vi "2.1调用.vi"(1 "数值 3":dbl, 2 "数值 2":dbl, 3 "数值":dbl) -> (0 "数值 4":dbl)   [LabVIEW 2017]
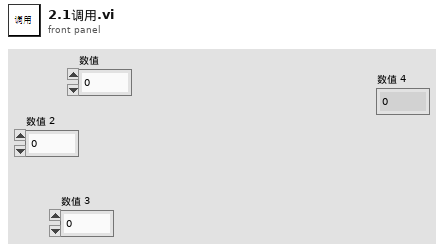
[diagram p1: front panel]
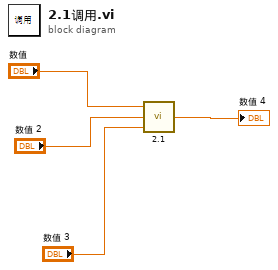
[diagram p0: block diagram]
diagram:
  n1 = call "2.1.vi"("数值 3"="数值 3", "数值 2"="数值 2", "数值"="数值") -> ("数值 4"=→"数值 4":dbl)
